vi "write_params.vi"(8 "error in (no error)":errorcluster caption="entrée d'erreur (pas d'erreur)", 10 "params":T1={"n_components"={"n_components_type"="None", "n_components_int"=0.0}, "alpha"=1.0, "max_iter"=1000.0, "tol"=1e-08, "fit_algorithm"="lars", "transform_algorithm"="omp", "transform_n_nonzero_coefs"={"transform_n_nonzero_coefs_type"="None", "transform_n_nonzero_coefs_int"=0.0}, "transform_alpha"=1.0, "n_jobs"=1.0, "code_init"=[], "dict_init"=[], "verbose"=FALSE, "split_sign"=FALSE, "random_state"=0.0, "positive_code"=FALSE, "positive_dict"=FALSE, "transform_max_iter"=1000.0}, 11 "DictionaryLearning en entrée":refnum<class "DictionaryLearning.lvclass">) -> (0 "error out":errorcluster caption="sortie d'erreur", 3 "DictionaryLearning en sortie":refnum<class "DictionaryLearning.lvclass">)   [LabVIEW 2020, in "DictionaryLearning.lvclass"]
uses:
  DictionaryLearning.lvclass
  Controls/dictionary_learning_params.ctl
  DictionaryLearning.lvclass/DictionaryLearning.ctl
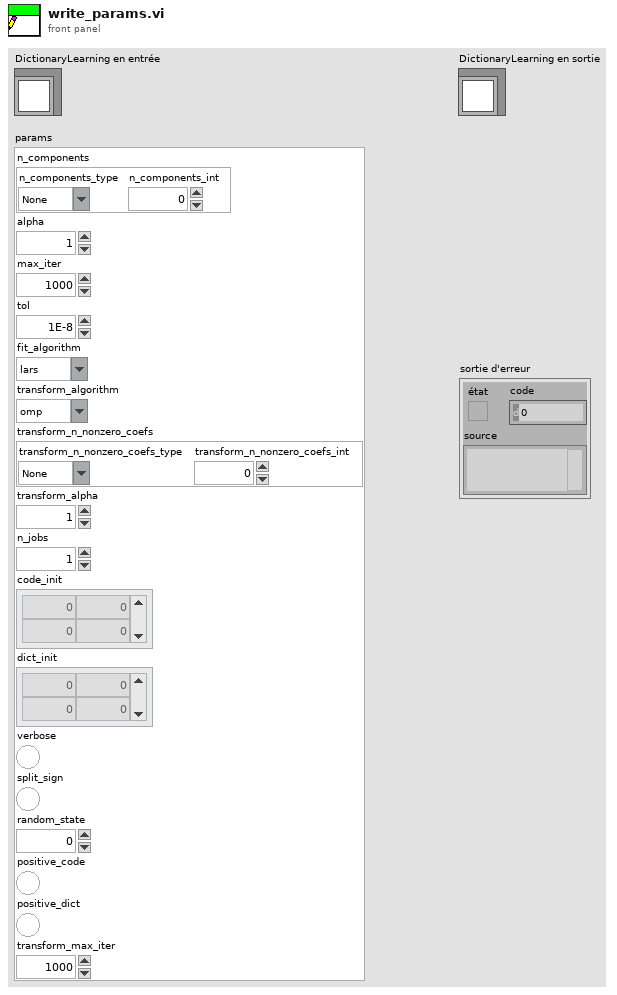
[diagram p1: front panel]
types:
  T1 = typedef "dictionary_learning_params.ctl" = cluster{"n_components":cluster{"n_components_type":string, "n_components_int":dbl}, "alpha":dbl, "max_iter":dbl, "tol":dbl, "fit_algorithm":string, "transform_algorithm":string, "transform_n_nonzero_coefs":cluster{"transform_n_nonzero_coefs_type":string, "transform_n_nonzero_coefs_int":dbl}, "transform_alpha":dbl, "n_jobs":dbl, "code_init":dbl[][], "dict_init":dbl[][], "verbose":bool, "split_sign":bool, "random_state":dbl, "positive_code":bool, "positive_dict":bool, "transform_max_iter":dbl}
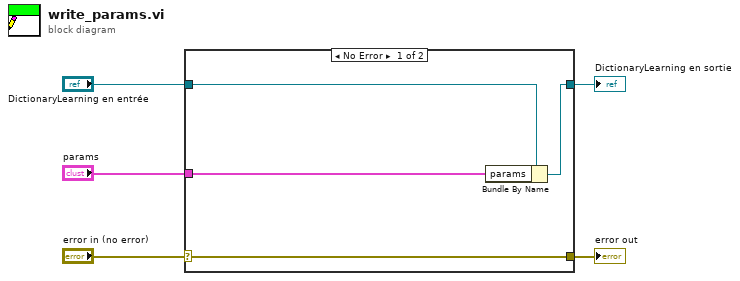
[diagram p0: block diagram]
diagram:
  n1 = case shown="No Error" "error in (no error)" {
    selector: "error in (no error)" -> [w9 w10]
    tunnel: [w9 w10] -> w4
    tunnel: [w8 w11] -> w2
    tunnel: "DictionaryLearning en entrée" -> [w6 w11]
    tunnel: "params" -> [w7 _]
    frame No Error {
      n2 = Bundle By Name(cluster=w6, "params"=w7) -> (w8:refnum<class "DictionaryLearning.lvclass">)
    }
    frame Error {
    }
  }
  "error out" <- w4
  "DictionaryLearning en sortie" <- w2
